vi "Publish.vi"(8 "error in (no error)":errorcluster, 10 "PublishRequest":refnum<class "PublishRequest.lvclass">, 11 "IMediator In":refnum<class "IMediator.lvclass">) -> (0 "error out":errorcluster, 3 "IMediator Out":refnum<class "IMediator.lvclass">)   [LabVIEW 2020, in "IMediator.lvlib" / "IMediator.lvclass"]
doc: "抽象方法\n发布"
uses:
  IMediator.lvclass
  PublishRequest/PublishRequest.lvclass
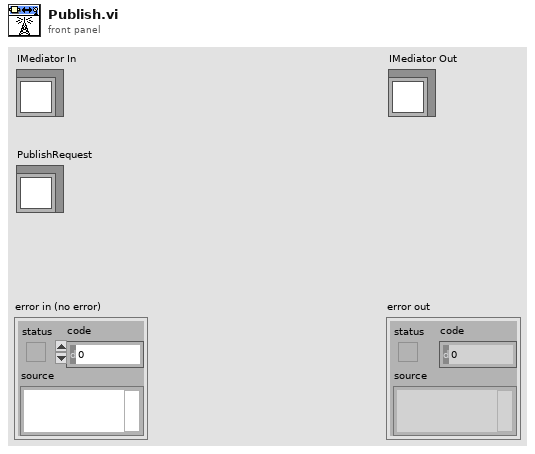
[diagram p1: front panel]
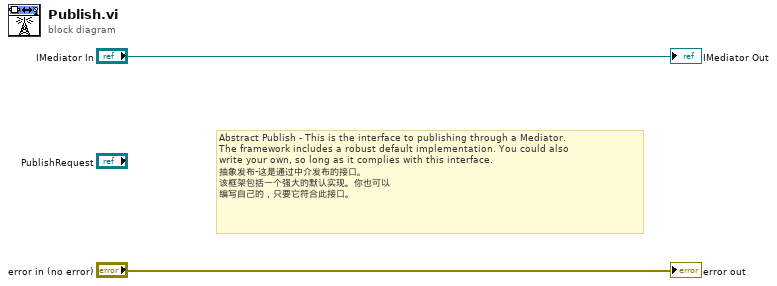
[diagram p0: block diagram]
diagram:
  # "Abstract Publish - This is the interface to publishing through a Mediator.\nThe framework includes a robust default implementation. You could also\nwrite your own, so long as it complies with this interface.\n抽象发布-这是通过中介发布的接口。\n该框架包括一个强大的默认实现。你也可以\n编写自己的，只要它符合此接口。"
  "error out" <- "error in (no error)"
  "IMediator Out" <- "IMediator In"
